vi "LED.vi"() -> ()   [LabVIEW 2023]
uses:
  <vilib>/Rock Robotics/WPI/Joystick/XBox Buttons Indexer.ctl
  <vilib>/Rock Robotics/WPI/DriverStation/WPI_DriverStationRobotMode2.ctl
  <vilib>/Rock Robotics/WPI/Utilities/WPI_GetSetVariantRefNum.vi
  Framework/Robot Global Data.vi
panel:
  in  "Color 8":u32(colorbox)=16711935
  in  "Color 7":u32(colorbox)=11403496
  in  "Color 6":u32(colorbox)=16860
  in  "Color 5":u32(colorbox)=65535
  in  "Color 4":u32(colorbox)=65280
  in  "Color 3":u32(colorbox)=16776960
  in  "Color 2":u32(colorbox)=16744448
  in  "Color":u32(colorbox)=16711680
  out "output array":u32[](array[numeric])
  out "Current Value":dbl
  out "error out":errorcluster
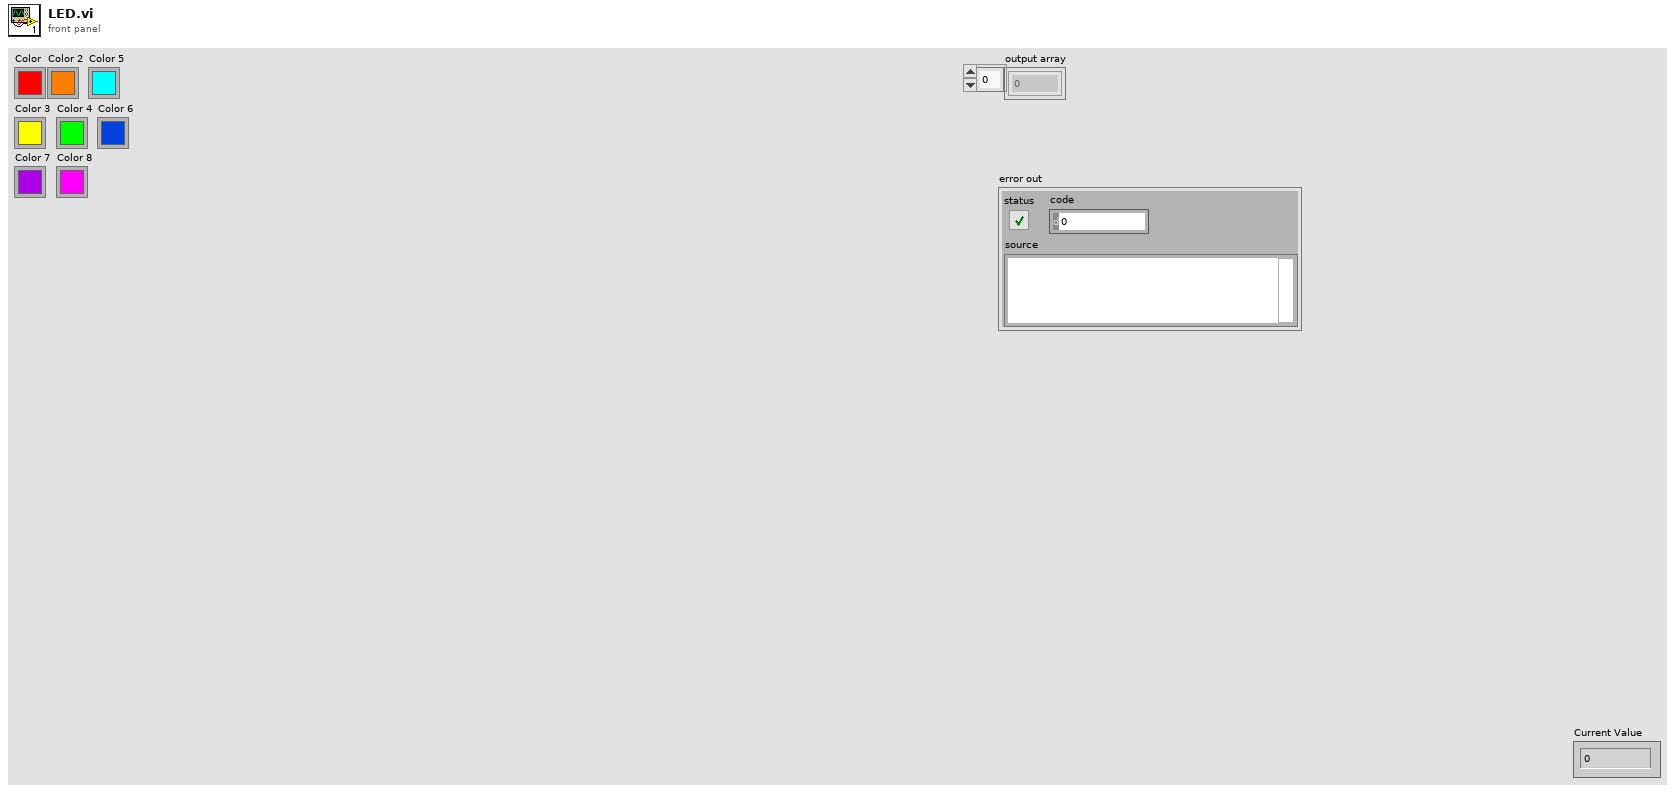
[diagram p1: front panel]
types:
  T1 = typedef "XBox Buttons Indexer.ctl" = enum16{"A", "B", "X", "Y", "Left Bumper", "Right Bumper", "Back", "Start", "Left Joystick", "Right Joystick"}
  T2 = typedef "WPI_DriverStationRobotMode2.ctl" = enum16{"Autonomous Disabled", "Autonomous Enabled", "Teleop Disabled", "Teleop Enabled", "Disconnected", "Finish", "Test Disabled", "Test Enabled", "Emergency Stopped"}
  T3 = typedef "WPI_DriverStationAllianceInfo.ctl" = enum16{"Red", "Blue", "Invalid"}
  T4 = enum16{"Station?", "Transfer", "Node 2", "Node 1", "Node 0"}
  T5 = typedef "WPI_DigitalInputDevRef.ctl" = cluster{"DevStatus":errorcluster, "DIO Channel":T6}
  T6 = typedef "FPGA_DIOChannel.ctl" = enum8{"DIO 0", "DIO 1", "DIO 2", "DIO 3", "DIO 4", "DIO 5", "DIO 6", "DIO 7", "DIO 8", "DIO 9", "DIO MXP 0", "DIO MXP 1", "DIO MXP 2", "DIO MXP 3", "DIO MXP 4", "DIO MXP 5", "DIO MXP 6", "DIO MXP 7", "DIO MXP 8", "DIO MXP 9", "DIO MXP 10", "DIO MXP 11", "DIO MXP 12", "DIO MXP 13", "DIO MXP 14", "DIO MXP 15", "SPI Port CS1", "SPI Port CS2", "SPI Port CS3", "SPI Port MISO", "SPI Port MOSI", "Invalid"}
  T7 = typedef "WPI_JoystickDevRef.ctl" = cluster{"Device":T8}
  T8 = typedef "WPI_JoystickDeviceEnum.ctl" = enum16{"USB 0", "USB 1", "USB 2", "USB 3", "USB 4", "USB 5"}
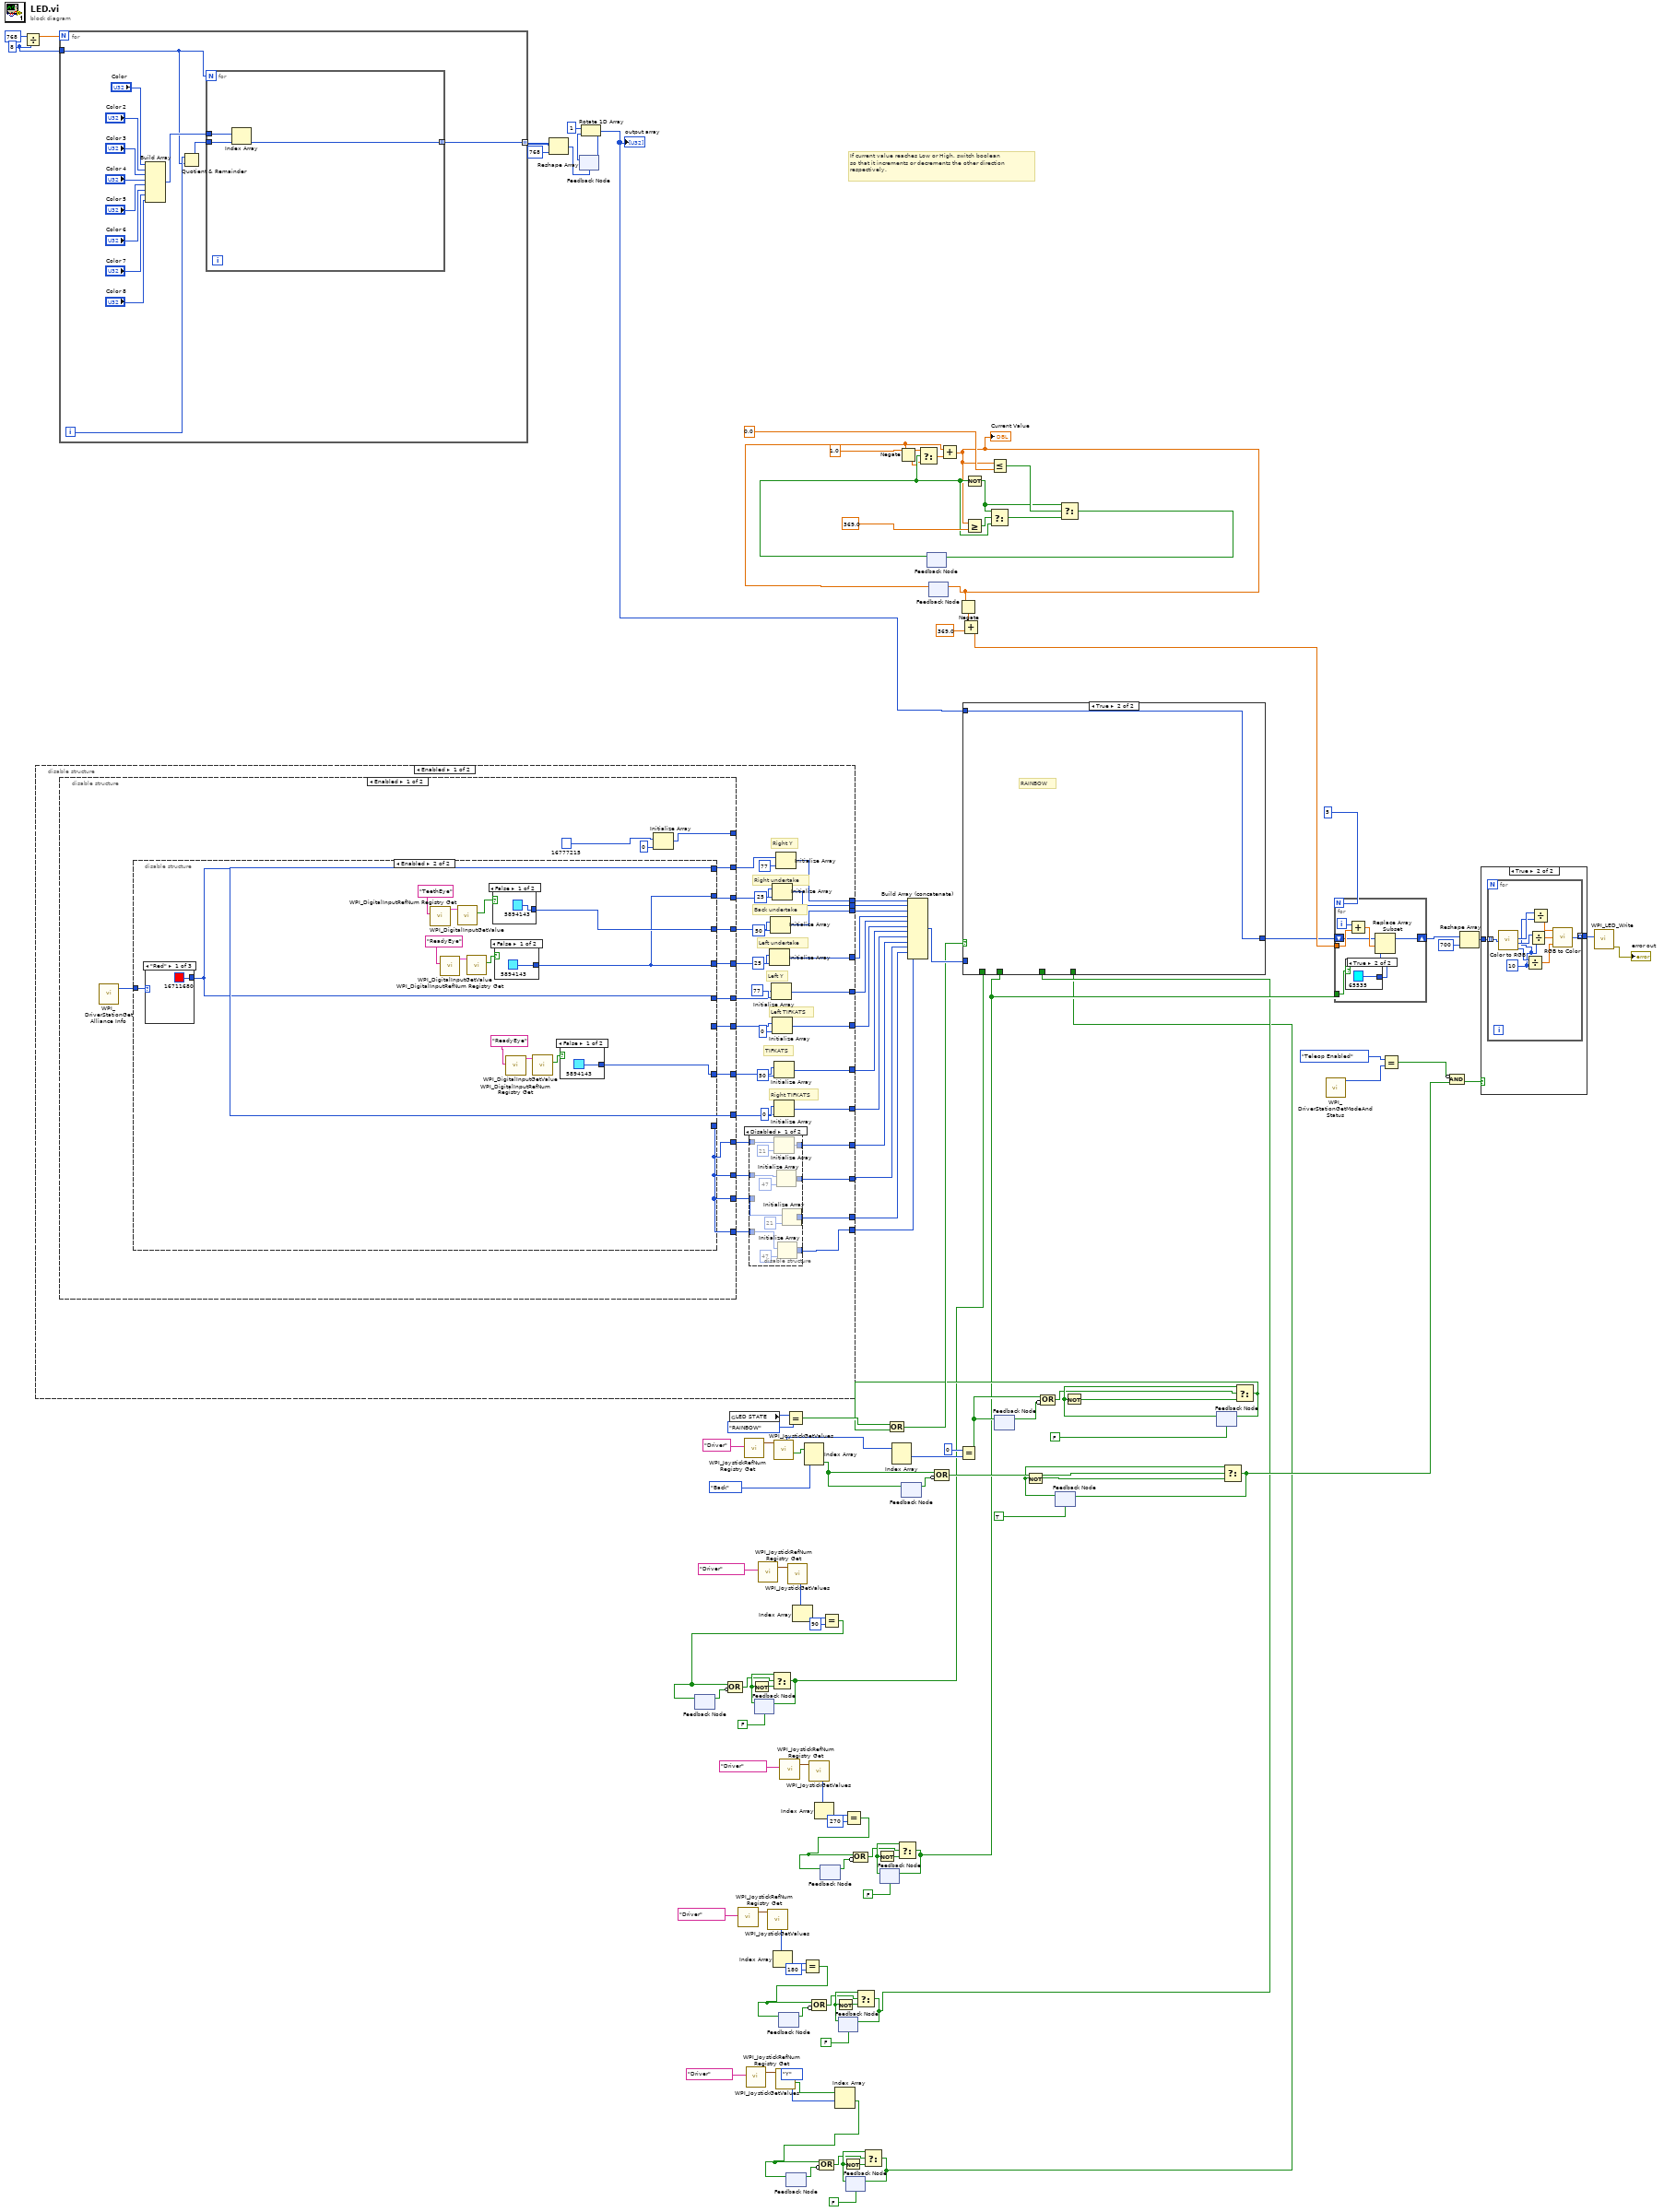
[diagram p0: block diagram]
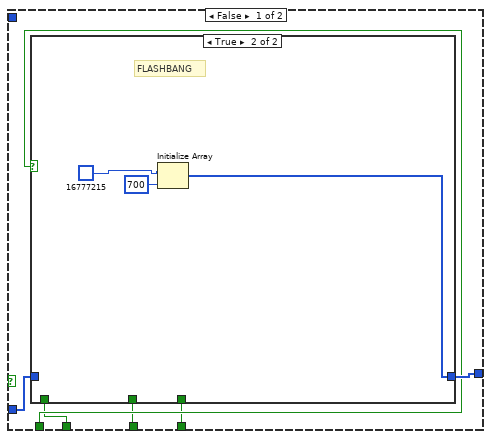
[diagram p3: hidden frame]
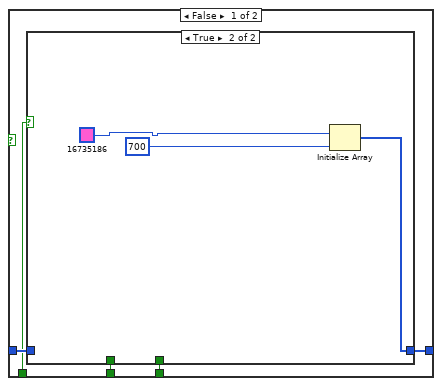
[diagram p4: hidden frame]
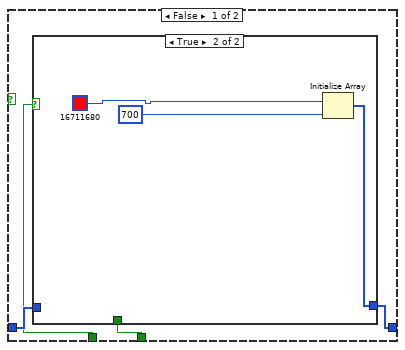
[diagram p5: hidden frame]
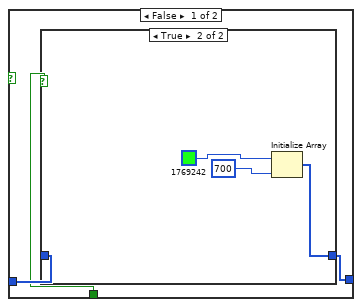
[diagram p6: hidden frame]
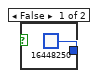
[diagram p8: hidden frame]
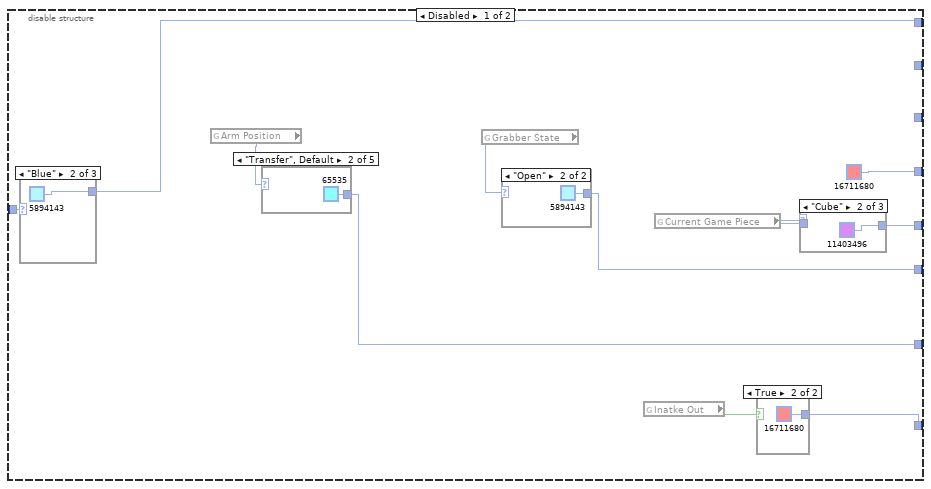
[diagram p10: hidden frame]
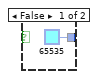
[diagram p11: hidden frame]
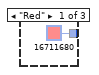
[diagram p12: hidden frame]
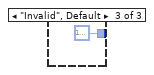
[diagram p13: hidden frame]
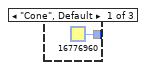
[diagram p14: hidden frame]
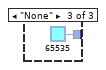
[diagram p15: hidden frame]
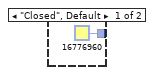
[diagram p16: hidden frame]
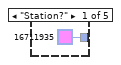
[diagram p17: hidden frame]
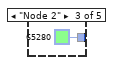
[diagram p18: hidden frame]
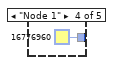
[diagram p19: hidden frame]
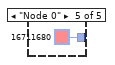
[diagram p20: hidden frame]
diagram:
  w98 = 8 ("y")
  # "If current value reaches Low or High, switch boolean\nso that it increments or decrements the other direction\nrespectively."
  n1 = Divide(x=768, y=w98) -> (x/y=w104:dbl)
  n2 = disable-structure shown="Enabled" {
    disable-tunnel: [w153 _] -> w120
    disable-tunnel: [w152 _] -> w119
    disable-tunnel: [w151 _] -> w83
    disable-tunnel: [w150 _] -> w118
    disable-tunnel: [w140 _] -> w80
    disable-tunnel: [w139 _] -> w4
    disable-tunnel: [w137 _] -> w2
    disable-tunnel: [w130 _] -> w82
    disable-tunnel: [w129 _] -> w84
    disable-tunnel: [w128 _] -> w81
    disable-tunnel: [w127 _] -> w3
    disable-tunnel: [w123 _] -> w1
    frame Enabled {
      # "Right TIFKATS"
      # "Left TIFKATS"
      # "TIFKATS"
      # "Left Y"
      # "Left undertake"
      # "Back undertake"
      # "Right undertake"
      # "Right Y"
      n3 = disable-structure shown="Enabled" {
        disable-tunnel: [w173 u32 16711680 ("Color")] -> w144
        disable-tunnel: [w177 u32 16775680 ("Color")] -> w142
        disable-tunnel: [w168 _] -> w138
        disable-tunnel: [w174 u32 6618880 ("Color")] -> w136
        disable-tunnel: [w176 u32 65535 ("Color")] -> w135
        disable-tunnel: [w175 u32 65535 ("Color")] -> w134
        disable-tunnel: [w175 u32 65535 ("Color")] -> w133
        disable-tunnel: [w167 u32 16711680 ("Color")] -> w132
        disable-tunnel: [w166 u32 65302 ("Color")] -> w131
        disable-tunnel: [w172 _] -> _
        disable-tunnel: [w168 _] -> w126
        disable-tunnel: [w168 _] -> w125
        disable-tunnel: [w168 _] -> w124
        frame Enabled {
          n4 = call <vilib>:"WPI_DriverStationGet Alliance Info.vi"() -> ("Alliance"=w171:T3)  [unwired: 6 in, 5 out]
          n5 = disable-structure shown="Enabled" {
            disable-tunnel: [w188 w216] -> w177
            disable-tunnel: [u32 16711680 ("Color") w208] -> w176
            disable-tunnel: [w186 w216] -> w175
            disable-tunnel: [w185 w204] -> w174
            disable-tunnel: [w184 _] -> w173
            disable-tunnel: w171 -> [w180 w217]
            disable-tunnel: [w179 _] -> w168
            disable-tunnel: [_ w212] -> w166
            disable-tunnel: [_ w208] -> w167
            frame Disabled {
              n6 = case shown="\"Blue\"" w180 {
                tunnel: [u32 16711680 ("Color") u32 5894143 ("Color") u32 16777225 ("Color")] -> w186
                frame "Red" {
                }
                frame "Blue" {
                }
                frame "Invalid", Default {
                }
              }
              n7 = global read "Robot Global Data.vi" "Arm Position"() -> (w183:T4)
              n8 = case shown="\"Transfer\", Default" w183 {
                tunnel: [u32 16711935 ("Color") u32 65535 ("Color") u32 65280 ("Color") u32 16776960 ("Color") u32 16711680 ("Color")] -> w185
                frame "Station?" {
                }
                frame "Transfer", Default {
                }
                frame "Node 2" {
                }
                frame "Node 1" {
                }
                frame "Node 0" {
                }
              }
              n9 = global read "Robot Global Data.vi" "Grabber State"() -> (w182:enum16{"Closed", "Open"})
              n10 = case shown="\"Open\"" w182 {
                tunnel: [u32 16776960 ("Color") u32 5894143 ("Color")] -> w184
                frame "Closed", Default {
                }
                frame "Open" {
                }
              }
              n11 = global read "Robot Global Data.vi" "Inatke Out"() -> (w178:bool)
              n12 = global read "Robot Global Data.vi" "Current Game Piece"() -> (w181:enum16{"Cone", "Cube", "None"})
              n13 = case shown="True" w178 {
                tunnel: [u32 65535 ("Color") u32 16711680 ("Color")] -> w179
                frame False {
                }
                frame True {
                }
              }
              n14 = case shown="\"Cube\"" w181 {
                tunnel: [u32 16776960 ("Color") u32 11403496 ("Color") u32 65535 ("Color")] -> w188
                tunnel: w181 -> [_ _ _]
                frame "Cone", Default {
                }
                frame "Cube" {
                }
                frame "None" {
                }
              }
            }
            frame Enabled {
              n15 = case shown="\"Red\"" w217 {
                tunnel: [u32 16711680 ("Color") u32 5894143 ("Color") u32 16777225 ("Color")] -> w216
                frame "Red" {
                }
                frame "Blue" {
                }
                frame "Invalid", Default {
                }
              }
              n16 = call <vilib>:"WPI_DigitalInputRefNum Registry Get.vi"("refnum name"="TeethEye") -> ("DigitalInputDevRef"=w215:T5)  [unwired: 9 in, 1 out]
              n17 = call <vilib>:"WPI_DigitalInputRefNum Registry Get.vi"("refnum name"="ReadyEye") -> ("DigitalInputDevRef"=w211:T5)  [unwired: 9 in, 1 out]
              n18 = call <vilib>:"WPI_DigitalInputGetValue.vi"("DigitalInputDevRef"=w215) -> ("Value"=w213:bool)  [unwired: 8 in, 2 out]
              n19 = call <vilib>:"WPI_DigitalInputGetValue.vi"("DigitalInputDevRef"=w211) -> ("Value"=w209:bool)  [unwired: 8 in, 2 out]
              n20 = case shown="False" w213 {
                tunnel: [u32 5894143 ("Color") u32 16747264 ("Color")] -> w212
                frame False {
                }
                frame True {
                }
              }
              n21 = case shown="False" w209 {
                tunnel: [u32 5894143 ("Color") u32 16747264 ("Color")] -> w208
                frame False {
                }
                frame True {
                }
              }
              n22 = call <vilib>:"WPI_DigitalInputRefNum Registry Get.vi"("refnum name"="ReadyEye") -> ("DigitalInputDevRef"=w207:T5)  [unwired: 9 in, 1 out]
              n23 = call <vilib>:"WPI_DigitalInputGetValue.vi"("DigitalInputDevRef"=w207) -> ("Value"=w205:bool)  [unwired: 8 in, 2 out]
              n24 = case shown="False" w205 {
                tunnel: [u32 5894143 ("Color") u32 16747264 ("Color")] -> w204
                frame False {
                }
                frame True {
                }
              }
            }
          }
          n25 = Initialize Array(u32 16777215 ("Color"), 0 ("dimension size")) -> (w172:u32[])
        }
        frame Disabled {
        }
      }
      n26 = disable-structure shown="Disabled" {
        disable-tunnel: [w165 _] -> w139
        disable-tunnel: w138 -> [w164 _]
        disable-tunnel: [w163 _] -> w137
        disable-tunnel: [w162 _] -> w127
        disable-tunnel: w126 -> [w161 _]
        disable-tunnel: w125 -> [w160 _]
        disable-tunnel: w124 -> [w159 _]
        disable-tunnel: [w158 _] -> w123
        frame Disabled {
          n27 = Initialize Array(w161, 21 ("dimension size")) -> (w165:u32[])
          n28 = Initialize Array(w160, 47 ("dimension size")) -> (w162:u32[])
          n29 = Initialize Array(w159, 47 ("dimension size")) -> (w158:u32[])
          n30 = Initialize Array(w164, 21 ("dimension size")) -> (w163:u32[])
        }
        frame Enabled {
        }
      }
      n31 = Initialize Array(w135, 25 ("dimension size")) -> (w129:u32[])
      n32 = Initialize Array(w131, 50 ("dimension size")) -> (w150:u32[])
      n33 = Initialize Array(w142, 77 ("dimension size")) -> (w151:u32[])
      n34 = Initialize Array(w132, 25 ("dimension size")) -> (w152:u32[])
      n35 = Initialize Array(w144, 0 ("dimension size")) -> (w128:u32[])
      n36 = Initialize Array(w136, 50 ("dimension size")) -> (w140:u32[])
      n37 = Initialize Array(w133, 0 ("dimension size")) -> (w130:u32[])
      n38 = Initialize Array(w134, 77 ("dimension size")) -> (w153:u32[])
    }
    frame Disabled {
    }
  }
  n39 = for {
    N: w104 -> [_]
    tunnel: [w237] -> w103 mode=indexing
    tunnel: w98 -> [w235]
    i -> [w236]
    n40 = Build Array("Color", "Color 2", "Color 3", "Color 4", "Color 5", "Color 6", "Color 7", "Color 8") -> (w239:u32[])
    n41 = Quotient & Remainder(x=w236, y=w235) -> (x-y*floor(x/y)=w238:i32)  [unwired: 1 out]
    n42 = for {
      N: w235 -> [_]
      tunnel: w239 -> [w250]
      tunnel: w238 -> [w249]
      tunnel: [w248] -> w237 mode=indexing
      n43 = Index Array(array=w250, index=w249) -> (element=w248:u32)
    }
  }
  n44 = Reshape Array(w103, 768 ("dimension size")) -> (w100:u32[])
  n45 = feedback #1(w100) -> (w101:u32[])
  n46 = Rotate 1D Array(1:w101, 2:1 ("n")) -> (0:w89:u32[])
  "output array" <- w89
  n47 = feedback-in #1(w89) -> ()
  n48 = feedback #2() -> (w43:bool)  [unwired: 1 in]
  n49 = global read "Robot Global Data.vi" "LED STATE"() -> (w79:enum16{"NORMAL", "RAINBOW"})
  n50 = call <vilib>:"WPI_JoystickRefNum Registry Get.vi"("refnum name"="Driver") -> ("JoystickDevRef"=w26:T7)  [unwired: 1 in, 9 out]
  n51 = call <vilib>:"WPI_JoystickRefNum Registry Get.vi"("refnum name"="Driver") -> ("JoystickDevRef"=w91:T7)  [unwired: 1 in, 9 out]
  n52 = call <vilib>:"WPI_JoystickRefNum Registry Get.vi"("refnum name"="Driver") -> ("JoystickDevRef"=w10:T7)  [unwired: 1 in, 9 out]
  n53 = feedback #3(FALSE) -> (w44:bool)
  n54 = Not(x=w44) -> (.not. x?=w45:bool)
  n55 = call <vilib>:"WPI_JoystickRefNum Registry Get.vi"("refnum name"="Driver") -> ("JoystickDevRef"=w50:T7)  [unwired: 1 in, 9 out]
  n56 = call <vilib>:"WPI_JoystickGetValues.vi"("JoystickDevRef"=w26) -> ("POVs"=w25:i16[])  [unwired: 6 in, 4 out]
  n57 = Index Array(array=w25) -> (element=w24:i16)  [unwired: 1 in]
  n58 = call <vilib>:"WPI_JoystickGetValues.vi"("JoystickDevRef"=w91) -> ("Buttons"=w90:bool[], "POVs"=w61:i16[])  [unwired: 6 in, 3 out]
  n59 = call <vilib>:"WPI_JoystickGetValues.vi"("JoystickDevRef"=w10) -> ("Buttons"=w7:bool[])  [unwired: 6 in, 4 out]
  n60 = feedback #4() -> (w19:bool)  [unwired: 1 in]
  n61 = call <vilib>:"WPI_JoystickRefNum Registry Get.vi"("refnum name"="Driver") -> ("JoystickDevRef"=w38:T7)  [unwired: 1 in, 9 out]
  n62 = Equal?(x=w79, y=enum16{"NORMAL", "RAINBOW"}."RAINBOW") -> (x = y?=w76:bool)
  n63 = feedback #5() -> (w12:bool)  [unwired: 1 in]
  n64 = call <vilib>:"WPI_JoystickGetValues.vi"("JoystickDevRef"=w50) -> ("POVs"=w49:i16[])  [unwired: 6 in, 4 out]
  n65 = Index Array(array=w49) -> (element=w48:i16)  [unwired: 1 in]
  n66 = Equal?(x=w24, y=i16 180) -> (x = y?=w17:bool)
  n67 = feedback-in #4(w17) -> ()
  n68 = Index Array(array=w90, index #2=XBox_Buttons_Indexer."Back" ("XBox Buttons")) -> (element #2=w71:bool)  [unwired: 1 in, 1 out]
  n69 = call <vilib>:"WPI_JoystickGetValues.vi"("JoystickDevRef"=w38) -> ("POVs"=w37:i16[])  [unwired: 6 in, 4 out]
  n70 = Compound Arithmetic op=OR(w17, invert w19) -> (w18:bool)
  n71 = Index Array(array=w37) -> (element=w36:i16)  [unwired: 1 in]
  n72 = feedback #6() -> (w31:bool)  [unwired: 1 in]
  n73 = Equal?(x=w48, y=i16 90) -> (x = y?=w41:bool)
  n74 = feedback-in #2(w41) -> ()
  n75 = Compound Arithmetic op=OR(w41, invert w43) -> (w42:bool)
  n76 = Select(t=w44, s=w42, f=w45) -> (s? t:f=w40:bool)
  n77 = feedback-in #3(w40) -> ()
  n78 = Index Array(array=w7, index #1=XBox_Buttons_Indexer."Y" ("XBox Buttons")) -> (element #1=w5:bool)  [unwired: 1 in, 1 out]
  n79 = feedback-in #5(w5) -> ()
  n80 = Compound Arithmetic op=OR(w5, invert w12) -> (w11:bool)
  n81 = feedback #7(FALSE) -> (w20:bool)
  n82 = Not(x=w20) -> (.not. x?=w21:bool)
  n83 = Equal?(x=w36, y=i16 270) -> (x = y?=w29:bool)
  n84 = feedback-in #6(w29) -> ()
  n85 = feedback #8(FALSE) -> (w13:bool)
  n86 = Not(x=w13) -> (.not. x?=w14:bool)
  n87 = Compound Arithmetic op=OR(w29, invert w31) -> (w30:bool)
  n88 = Select(t=w20, s=w18, f=w21) -> (s? t:f=w16:bool)
  n89 = feedback-in #7(w16) -> ()
  n90 = Select(t=w13, s=w11, f=w14) -> (s? t:f=w8:bool)
  n91 = feedback-in #8(w8) -> ()
  n92 = feedback #9(FALSE) -> (w32:bool)
  n93 = Not(x=w32) -> (.not. x?=w33:bool)
  n94 = Index Array(array=w61) -> (element #1=w60:i16)  [unwired: 2 in, 1 out]
  n95 = Select(t=w32, s=w30, f=w33) -> (s? t:f=w28:bool)
  n96 = feedback-in #9(w28) -> ()
  n97 = feedback-in #10(w71) -> ()
  n98 = feedback #10() -> (w72:bool)  [unwired: 1 in]
  n99 = Build Array (concatenate)(w120, w119, w118, w84, w83, w81, w80, w82, w4, w3, w2, w1) -> (w87:u32[])
  n100 = feedback #11() -> (w108:bool)  [unwired: 1 in]
  n101 = feedback #12() -> (w107:dbl)  [unwired: 1 in]
  n102 = Negate(x=w107) -> (-x=w106:dbl)
  n103 = Select(t=1.0 ("Increment"), s=w108, f=w106) -> (s? t:f=w115:dbl)
  n104 = Compound Arithmetic op=OR(w71, invert w72) -> (w70:bool)
  n105 = Add(x=w107, y=w115) -> (x+y=w96:dbl)
  "Current Value" <- w96
  n106 = feedback-in #12(w96) -> ()
  n107 = Negate(x=w96) -> (-x=w95:dbl)
  n108 = Equal?(x=i16 0, y=w60) -> (x = y?=w53:bool)
  n109 = Add(x=w95, y=369.0) -> (x+y=w94:dbl)
  n110 = Not(x=w108) -> (.not. x?=w110:bool)
  n111 = Greater Or Equal?(x=w96, y=369.0 ("High")) -> (x >= y?=w114:bool)
  n112 = Less Or Equal?(x=w96, y=0.0 ("Low")) -> (x <= y?=w111:bool)
  n113 = Select(t=w110, s=w114, f=w108) -> (s? t:f=w113:bool)
  n114 = feedback #13() -> (w54:bool)  [unwired: 1 in]
  n115 = feedback-in #13(w53) -> ()
  n116 = Compound Arithmetic op=OR(w53, invert w54) -> (w52:bool)
  n117 = feedback #14(TRUE) -> (w62:bool)
  n118 = Not(x=w62) -> (.not. x?=w63:bool)
  n119 = Select(t=w110, s=w111, f=w113) -> (s? t:f=w109:bool)
  n120 = feedback-in #11(w109) -> ()
  n121 = feedback #15(FALSE) -> (w56:bool)
  n122 = Not(x=w56) -> (.not. x?=w57:bool)
  n123 = Select(t=w62, s=w70, f=w63) -> (s? t:f=w68:bool)
  n124 = feedback-in #14(w68) -> ()
  n125 = Select(t=w56, s=w52, f=w57) -> (s? t:f=w55:bool)
  n126 = Or(x=w76, y=w55) -> (x .or. y?=w77:bool)
  n127 = case shown="True" w77 {
    tunnel: w89 -> [_ w282]
    tunnel: [w256 w282] -> w88
    tunnel: w87 -> [w255 _]
    tunnel: w40 -> [w254 _]
    tunnel: w28 -> [w253 _]
    tunnel: w16 -> [w252 _]
    tunnel: w8 -> [w251 _]
    frame False {
      n128 = case shown="True" w254 {
        tunnel: [w261 w279] -> w256
        tunnel: w255 -> [w260 _]
        tunnel: w253 -> [w259 _]
        tunnel: w252 -> [w258 _]
        tunnel: w251 -> [w257 _]
        frame False {
          n129 = case shown="True" w259 {
            tunnel: [w265 w276] -> w261
            tunnel: w260 -> [w264 _]
            tunnel: w258 -> [w263 _]
            tunnel: w257 -> [w262 _]
            frame False {
              n130 = case shown="True" w263 {
                tunnel: [w267 w273] -> w265
                tunnel: w264 -> [w268 _]
                tunnel: w262 -> [w266 _]
                frame False {
                  n131 = case shown="True" w266 {
                    tunnel: w268 -> [w269 _]
                    tunnel: [w269 w270] -> w267
                    frame False {
                      # "NORMAL"
                    }
                    frame True {
                      n132 = Initialize Array(u32 1769242 ("Color"), 700 ("dimension size")) -> (w270:u32[])
                    }
                  }
                }
                frame True {
                  n133 = Initialize Array(u32 16711680 ("Color"), 700 ("dimension size")) -> (w273:u32[])
                }
              }
            }
            frame True {
              n134 = Initialize Array(u32 16735186 ("Color"), 700 ("dimension size")) -> (w276:u32[])
            }
          }
        }
        frame True {
          # "FLASHBANG"
          n135 = Initialize Array(u32 16777215 ("Color"), 700 ("dimension size")) -> (w279:u32[])
        }
      }
    }
    frame True {
      # "RAINBOW"
    }
  }
  n136 = feedback-in #15(w55) -> ()
  n137 = call <vilib>:"WPI_DriverStationGetModeAndStatus.vi"() -> ("Robot Mode"=w65:T2)  [unwired: 10 in, 1 out]
  n138 = for {
    N: 5 -> [_]
    tunnel: w94 -> [w288]
    shift-right: [w284] -> w86
    shift-left: w88 -> [w285]
    tunnel: w28 -> [w283]
    i -> [w287]
    n139 = case shown="True" w283 {
      tunnel: [u32 16448250 ("Color") u32 65535 ("Color")] -> w289
      frame False {
      }
      frame True {
      }
    }
    n140 = Add(x=w287, y=w288) -> (x+y=w286:dbl)
    n141 = Replace Array Subset(array=w285, new element=w289, index=w286) -> (w284:u32[])
  }
  n142 = Equal?(x=WPI_DriverStationRobotMode2."Teleop Enabled" ("Robot Mode"), y=w65) -> (x = y?=w64:bool)
  n143 = Compound Arithmetic op=AND(invert w64, w68) -> (w67:bool)
  n144 = Reshape Array(w86, 700 ("dimension size")) -> (w74:u32[])
  n145 = case shown="True" w67 {
    tunnel: [w292 w294] -> w75
    tunnel: w74 -> [w292 w293]
    frame False {
    }
    frame True {
      n146 = for {
        tunnel: [w302] -> w294 mode=indexing
        tunnel: w293 -> [w303] mode=indexing
        w295 = u8 10 ("y")
        n147 = call <vilib>:"Color to RGB.vi"("Color"=w303) -> ("R"=w298:u8, "G"=w296:u8, "B"=w297:u8)  [unwired: 1 out]
        n148 = Divide(x=w297, y=w295) -> (x/y=w301:dbl)
        n149 = Divide(x=w296, y=w295) -> (x/y=w300:dbl)
        n150 = Divide(x=w298, y=w295) -> (x/y=w299:dbl)
        n151 = call <vilib>:"RGB to Color.vi"("B"=w301, "G"=w300, "R"=w299) -> ("Color"=w302:u32)
      }
    }
  }
  n152 = call <vilib>:"WPI_LED_Write.vi"("Color Array"=w75) -> ("error out"=→"error out":errorcluster)  [unwired: 10 in]
